vi "xnet_init.vi"() -> (0 "Error out B":errorcluster, 1 "XNET session B":refnum<k21>, 2 "Error out A":errorcluster, 3 "XNET session A":refnum<k21>)   [LabVIEW 2017]
uses:
  <vilib>/xnet/xnet.llb/XNET Create Session (Frame Input Stream).vi
  <resource>/objmgr/xnet.rc
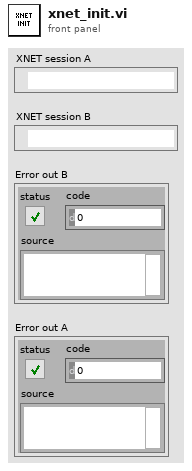
[diagram p1: front panel]
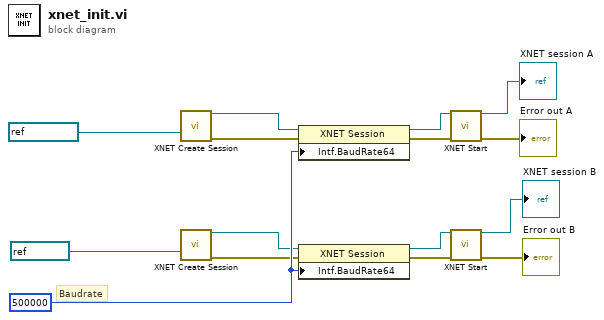
[diagram p0: block diagram]
diagram:
  w13 = 500000
  # "Baudrate"
  n1 = call-poly <vilib>:"XNET Create Session.vi"("interface"=refnum<k21> "CAN2" ("XNET Interface")) -> ("session out"=w11:refnum<k21>, "error out"=w12:errorcluster)  [unwired: 13 in]
  n2 = call-poly <vilib>:"XNET Create Session.vi"("interface"=refnum<k21> "CAN3" ("XNET Interface")) -> ("session out"=w8:refnum<k21>, "error out"=w7:errorcluster)  [unwired: 13 in]
  n3 = property class="XNET Session"(reference=w11, error in=w12, "Intf.BaudRate64"=w13) -> (reference out=w10:refnum<k21>, error out=w9:errorcluster)
  n4 = property class="XNET Session"(reference=w8, error in=w7, "Intf.BaudRate64"=w13) -> (reference out=w6:refnum<k21>, error out=w5:errorcluster)
  n5 = call <vilib>:"XNET Start.vi"("session in"=w10, "error in (no error)"=w9) -> ("session out"=→"XNET session A":refnum<k21>, "error out"=→"Error out A":errorcluster)  [unwired: 12 in]
  n6 = call <vilib>:"XNET Start.vi"("session in"=w6, "error in (no error)"=w5) -> ("session out"=→"XNET session B":refnum<k21>, "error out"=→"Error out B":errorcluster)  [unwired: 12 in]
